vi "hmi_negative_feedback.vi"(8 "error in (no error)":errorcluster, 9 "f_button":string="No", 10 "t_button":string="Yes", 11 "dialog_text":string="Action failed, show error?") -> (0 "error out":errorcluster)   [LabVIEW 2015, in "lv-build-interface.lvlib"]
uses:
  lv-build-interface.lvlib
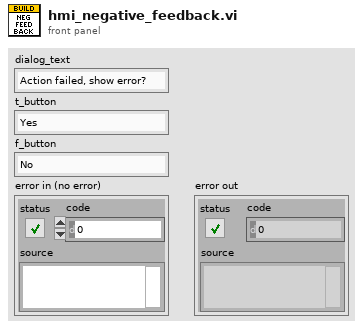
[diagram p1: front panel]
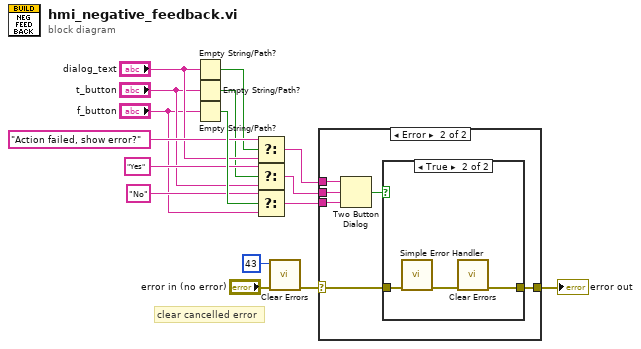
[diagram p0: block diagram]
diagram:
  # "clear cancelled error"
  n1 = Empty String/Path?(string/path="dialog_text") -> (empty?=w9:bool)
  n2 = Empty String/Path?(string/path="t_button") -> (empty?=w6:bool)
  n3 = Empty String/Path?(string/path="f_button") -> (empty?=w12:bool)
  n4 = Select(t="Action failed, show error?" ("dialog_text"), s=w9, f="dialog_text") -> (s? t:f=w1:string)
  n5 = Select(t="Yes" ("t_button"), s=w6, f="t_button") -> (s? t:f=w2:string)
  n6 = Select(t="No" ("f_button"), s=w12, f="f_button") -> (s? t:f=w3:string)
  n7 = call <vilib>:"Clear Errors.vi"("error in (no error)"="error in (no error)", "specific error code to clear (0: all)"=43) -> ("error out"=w14:errorcluster)  [unwired: 4 in, 1 out]
  n8 = case shown="Error" w14 {
    selector: w14 -> [w17 w20]
    tunnel: w1 -> [_ w23]
    tunnel: w2 -> [_ w22]
    tunnel: w3 -> [_ w21]
    tunnel: [w17 w18] -> w16
    frame No Error {
    }
    frame Error {
      n9 = Two Button Dialog(message=w23, 1:w21, 2:w22) -> (T button?=w19:bool)
      n10 = case shown="True" w19 {
        tunnel: w20 -> [w24 w27]
        tunnel: [w24 w25] -> w18
        frame False {
        }
        frame True {
          n11 = call <vilib>:"Simple Error Handler.vi"("error in (no error)"=w27) -> ("error out"=w26:errorcluster)  [unwired: 4 in, 4 out]
          n12 = call <vilib>:"Clear Errors.vi"("error in (no error)"=w26) -> ("error out"=w25:errorcluster)  [unwired: 5 in, 1 out]
        }
      }
    }
  }
  "error out" <- w16
